vi "2039_BackTalonOut.vi"(5 "Throttle Ramp Rate (percent/s)":dbl, 6 "Invert Stop Condition":bool, 7 "Speed to run motor (will be negated)":dbl=0.2, 8 "error in (no error)":errorcluster, 9 "DIO Ref Name":string="My DI RefNum", 10 "Brake":bool=TRUE, 11 "CAN Talon SRX Ref":T1={"DeviceStatus"={"status"=FALSE, "code"=0, "source"=""}, "Type"=enum."PWM", "PWM"={"PWM Channel"=enum."PWM 1", "DeadBand"={"Name"="", "maxPositivePwm"=0, "minPositivePwm"=0, "centerPwm"=0, "maxNegativePwm"=0, "minNegativePwm"=0, "angularRange"=0}}, "CAN"={"Device Number"=0, "Control Mode"=enum."Percent VBus", "Semaphore"=refnum, "Max Vout"=12.0, "TalonSRX Control Mode"=enum."Percent VBus"}, "Invert"=FALSE}) -> (0 "error out":errorcluster, 3 "CAN Talon SRX Ref Out":T1={"DeviceStatus"={"status"=FALSE, "code"=0, "source"=""}, "Type"=enum."PWM", "PWM"={"PWM Channel"=enum."PWM 1", "DeadBand"={"Name"="", "maxPositivePwm"=0, "minPositivePwm"=0, "centerPwm"=0, "maxNegativePwm"=0, "minNegativePwm"=0, "angularRange"=0}}, "CAN"={"Device Number"=0, "Control Mode"=enum."Percent VBus", "Semaphore"=refnum, "Max Vout"=12.0, "TalonSRX Control Mode"=enum."Percent VBus"}, "Invert"=FALSE})   [LabVIEW 2015]
uses:
  <vilib>/Rock Robotics/WPI/MotorControl/WPI_MotorControlDeviceRef.ctl
  <vilib>/Rock Robotics/WPI/MotorControl/WPI_MotorControlType.ctl
  <vilib>/Rock Robotics/SystemInterfaces/DIO/FPGA_DIOPWMChannel.ctl
  <vilib>/Rock Robotics/WPI/PWM/WPI_PWMDeadband.ctl
  <vilib>/Rock Robotics/WPI/CAN/Jaguar/SubVIs/WPI_CANJaguar_ControlMode.ctl
  <vilib>/Rock Robotics/WPI/CAN/TalonSRX/WPI_CANTalonSRX_APIControlMode.ctl
  <vilib>/Rock Robotics/WPI/CAN/TalonSRX/WPI_CANTalonSRX_BrakeOverride.ctl
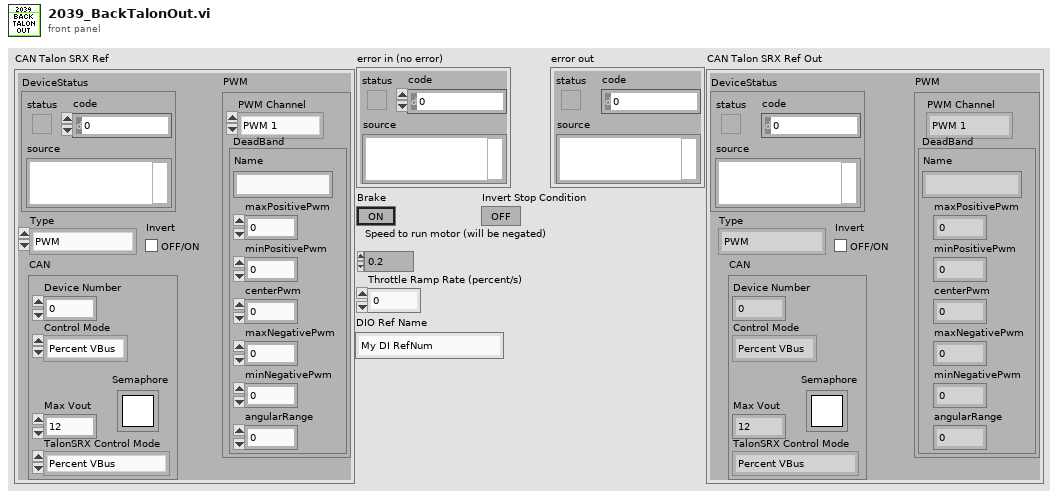
[diagram p1: front panel]
types:
  T1 = typedef "WPI_MotorControlDeviceRef.ctl" = cluster{"DeviceStatus":errorcluster, "Type":T2, "PWM":cluster{"PWM Channel":T3, "DeadBand":T4}, "CAN":cluster{"Device Number":u8, "Control Mode":T5, "Semaphore":T6, "Max Vout":dbl, "TalonSRX Control Mode":T7}, "Invert":bool}
  T2 = typedef "WPI_MotorControlType.ctl" = enum16{"PWM", "CAN", "CANTalonSRX"}
  T3 = typedef "FPGA_DIOPWMChannel.ctl" = enum8{"PWM 0", "PWM 1", "PWM 2", "PWM 3", "PWM 4", "PWM 5", "PWM 6", "PWM 7", "PWM 8", "PWM 9", "PWM MXP 0", "PWM MXP 1", "PWM MXP 2", "PWM MXP 3", "PWM MXP 4", "PWM MXP 5", "PWM MXP 6", "PWM MXP 7", "PWM MXP 8", "PWM MXP 9", "Invalid"}
  T4 = typedef "WPI_PWMDeadband.ctl" = cluster{"Name":string, "maxPositivePwm":i32, "minPositivePwm":i32, "centerPwm":i32, "maxNegativePwm":i32, "minNegativePwm":i32, "angularRange":u16}
  T5 = typedef "WPI_CANJaguar_ControlMode.ctl" = enum8{"Percent VBus", "Current", "Speed", "Position", "Voltage"}
  T6 = typedef "Semaphore RefNum" = refnum<k1>
  T7 = typedef "WPI_CANTalonSRX_APIControlMode.ctl" = enum8{"Percent VBus", "Speed", "Position", "Slave", "Unchanged / Invalid", "Voltage Compensation", "Current", "Motion Profile"}
  T8 = typedef "WPI_CANTalonSRX_BrakeOverride.ctl" = enum8{"No Override", "Override to Coast", "Override to Brake"}
  T9 = typedef "WPI_DigitalInputDevRef.ctl" = cluster{"DevStatus":errorcluster, "DIO Channel":T10}
  T10 = typedef "FPGA_DIOChannel.ctl" = enum8{"DIO 0", "DIO 1", "DIO 2", "DIO 3", "DIO 4", "DIO 5", "DIO 6", "DIO 7", "DIO 8", "DIO 9", "DIO MXP 0", "DIO MXP 1", "DIO MXP 2", "DIO MXP 3", "DIO MXP 4", "DIO MXP 5", "DIO MXP 6", "DIO MXP 7", "DIO MXP 8", "DIO MXP 9", "DIO MXP 10", "DIO MXP 11", "DIO MXP 12", "DIO MXP 13", "DIO MXP 14", "DIO MXP 15", "Invalid"}
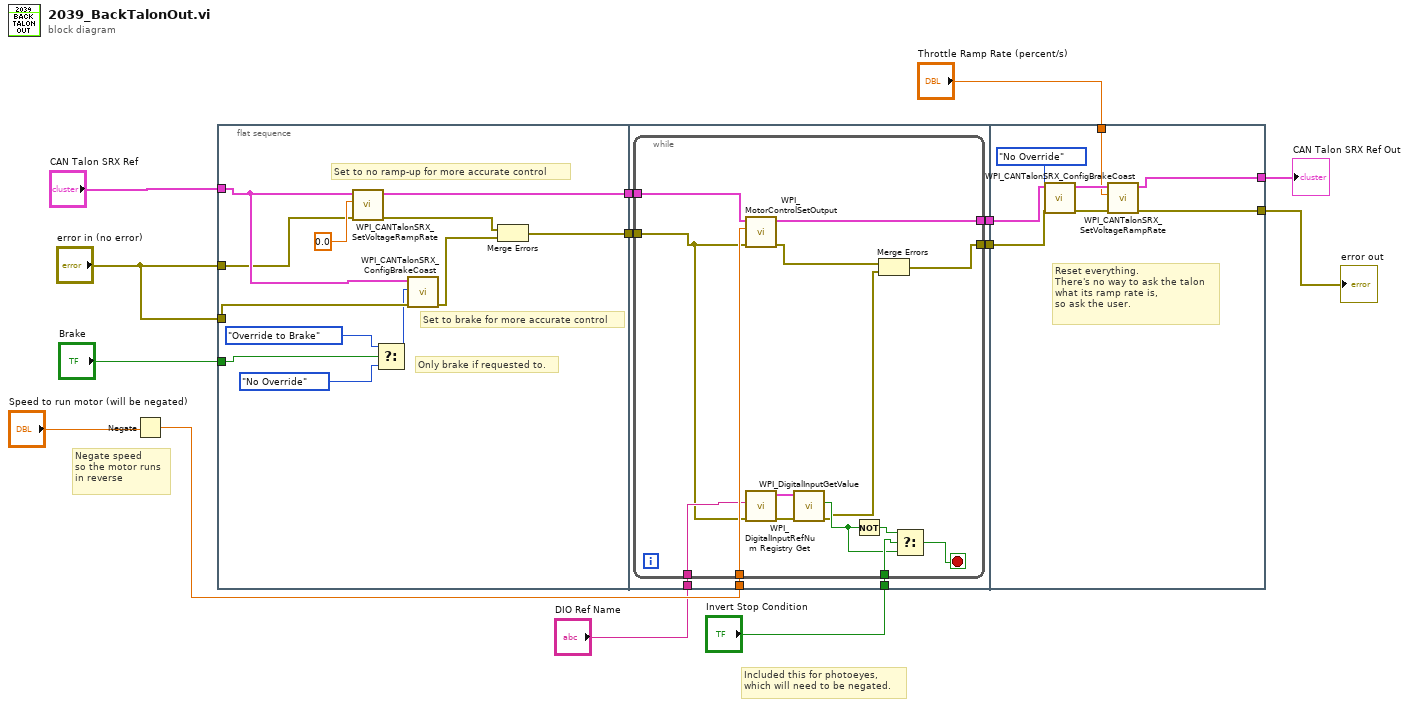
[diagram p0: block diagram]
diagram:
  # "Included this for photoeyes,\nwhich will need to be negated."
  # "Negate speed\nso the motor runs\nin reverse"
  n1 = Negate(x="Speed to run motor (will be negated)") -> (-x=w8:dbl)
  n2 = flat-sequence {
    tunnel: "CAN Talon SRX Ref" -> [w25]
    tunnel: "error in (no error)" -> [w24]
    tunnel: "error in (no error)" -> [w23]
    tunnel: "Brake" -> [w20]
    tunnel: [w16] -> w11
    tunnel: [w15] -> w10
    tunnel: w11 -> [w30]
    tunnel: w10 -> [w32]
    tunnel: "Invert Stop Condition" -> [w33]
    tunnel: w8 -> [w31]
    tunnel: [w29] -> w5
    tunnel: [w28] -> w4
    tunnel: "DIO Ref Name" -> [w27]
    tunnel: "Throttle Ramp Rate (percent/s)" -> [w53]
    tunnel: w5 -> [w52]
    tunnel: w4 -> [w50]
    tunnel: [w49] -> w3
    tunnel: [w48] -> w2
    frame #0 {
      # "Only brake if requested to."
      # "Set to brake for more accurate control"
      # "Set to no ramp-up for more accurate control"
      n3 = call <vilib>:"WPI_CANTalonSRX_SetVoltageRampRate.vi"("error in (no error)"=w24, "Throttle Ramp Rate (percent/s)"=0.0, "CAN Talon SRX Ref"=w25) -> ("error out"=w18:errorcluster, "CAN Talon SRX Ref"=w15:T1)  [unwired: 7 in]
      n4 = Select(t=WPI_CANTalonSRX_BrakeOverride."Override to Brake" ("Brake / Coast Mode"), s=w20, f=WPI_CANTalonSRX_BrakeOverride."No Override" ("Brake / Coast Mode")) -> (s? t:f=w19:T8)
      n5 = call <vilib>:"WPI_CANTalonSRX_ConfigBrakeCoast.vi"("error in (no error)"=w23, "Brake / Coast Mode"=w19, "CAN Talon SRX Ref"=w25) -> ("error out"=w17:errorcluster)  [unwired: 7 in, 1 out]
      n6 = Merge Errors(w18, w17) -> (w16:errorcluster)
    }
    frame #1 {
      n7 = while {
        tunnel: w33 -> [w46]
        tunnel: w32 -> [w44]
        tunnel: w31 -> [w43]
        tunnel: w30 -> [w40]
        tunnel: [w42] -> w29
        tunnel: [w34] -> w28
        tunnel: w27 -> [w41]
        stop <- w45 stop-if-true
        n8 = call <vilib>:"WPI_MotorControlSetOutput.vi"("error in (no error)"=w40, "Output"=w43, "MotorControlDevRef"=w44) -> ("error out"=w36:errorcluster, "MotorControlDevRef"=w42:T1)  [unwired: 6 in, 1 out]
        n9 = call <vilib>:"WPI_DigitalInputRefNum Registry Get.vi"("error in (no error)"=w40, "refnum name"=w41) -> ("error out"=w39:errorcluster, "DigitalInputDevRef"=w38:T9)  [unwired: 8 in]
        n10 = call <vilib>:"WPI_DigitalInputGetValue.vi"("error in (no error)"=w39, "DigitalInputDevRef"=w38) -> ("error out"=w35:errorcluster, "Value"=w37:bool)  [unwired: 7 in, 1 out]
        n11 = Not(x=w37) -> (.not. x?=w47:bool)
        n12 = Merge Errors(w36, w35) -> (w34:errorcluster)
        n13 = Select(t=w47, s=w46, f=w37) -> (s? t:f=w45:bool)
      }
    }
    frame #2 {
      # "Reset everything.\nThere's no way to ask the talon\nwhat its ramp rate is,\nso ask the user."
      n14 = call <vilib>:"WPI_CANTalonSRX_ConfigBrakeCoast.vi"("error in (no error)"=w50, "Brake / Coast Mode"=WPI_CANTalonSRX_BrakeOverride."No Override", "CAN Talon SRX Ref"=w52) -> ("error out"=w55:errorcluster, "CAN Talon SRX Ref"=w54:T1)  [unwired: 7 in]
      n15 = call <vilib>:"WPI_CANTalonSRX_SetVoltageRampRate.vi"("error in (no error)"=w55, "Throttle Ramp Rate (percent/s)"=w53, "CAN Talon SRX Ref"=w54) -> ("error out"=w49:errorcluster, "CAN Talon SRX Ref"=w48:T1)  [unwired: 7 in]
    }
  }
  "error out" <- w3
  "CAN Talon SRX Ref Out" <- w2
